vi "daq.vi"(5 "data queue 1":refnum<queue>, 7 "data queue 2":refnum<queue>, 8 "error in":errorcluster, 9 "finished late":bool, 10 "vars runtime":T2[](array[typedef])=[{"t wait"=1000, "t stim"=0, "t square"=0, "t digStimOne"=0, "t digStimTwo"=0, "t rew"=0, "t onset"=10000, "n stim"=0, "n hit"=0, "n miss"=0, "n catch"=0, "n reject"=0, "n false alarm"=0, "stim amp"=0.0, "stim idx"=0, "next temp"=32.0, "catch"=FALSE, "stimulus"=FALSE, "reward given"=FALSE, "penalty given"=FALSE, "lick"=FALSE, "next reward"=FALSE, "penalty"=FALSE, "backlight"=FALSE, "square"=FALSE, "digStimOne"=FALSE, "digStimTwo"=FALSE, "first run?"=TRUE, "timeout"=FALSE, "free reward"=FALSE, "pairing"=FALSE, "d stim"=0, "d square"=0, "n rew"=0, "t penalty"=0}, {"t wait"=1000, "t stim"=0, "t square"=0, "t digStimOne"=0, "t digStimTwo"=0, "t rew"=0, "t onset"=10000, "n stim"=0, "n hit"=0, "n miss"=0, "n catch"=0, "n reject"=0, "n false alarm"=0, "stim amp"=0.0, "stim idx"=0, "next temp"=32.0, "catch"=FALSE, "stimulus"=FALSE, "reward given"=FALSE, "penalty given"=FALSE, "lick"=FALSE, "next reward"=FALSE, "penalty"=FALSE, "backlight"=FALSE, "square"=FALSE, "digStimOne"=FALSE, "digStimTwo"=FALSE, "first run?"=TRUE, "timeout"=FALSE, "free reward"=FALSE, "pairing"=FALSE, "d stim"=0, "d square"=0, "n rew"=0, "t penalty"=0}, {"t wait"=1000, "t stim"=0, "t square"=0, "t digStimOne"=0, "t digStimTwo"=0, "t rew"=0, "t onset"=10000, "n stim"=0, "n hit"=0, "n miss"=0, "n catch"=0, "n reject"=0, "n false alarm"=0, "stim amp"=0.0, "stim idx"=0, "next temp"=32.0, "catch"=FALSE, "stimulus"=FALSE, "reward given"=FALSE, "penalty given"=FALSE, "lick"=FALSE, "next reward"=FALSE, "penalty"=FALSE, "backlight"=FALSE, "square"=FALSE, "digStimOne"=FALSE, "digStimTwo"=FALSE, "first run?"=TRUE, "timeout"=FALSE, "free reward"=FALSE, "pairing"=FALSE, "d stim"=0, "d square"=0, "n rew"=0, "t penalty"=0}, {"t wait"=1000, "t stim"=0, "t square"=0, "t digStimOne"=0, "t digStimTwo"=0, "t rew"=0, "t onset"=10000, "n stim"=0, "n hit"=0, "n miss"=0, "n catch"=0, "n reject"=0, "n false alarm"=0, "stim amp"=0.0, "stim idx"=0, "next temp"=32.0, "catch"=FALSE, "stimulus"=FALSE, "reward given"=FALSE, "penalty given"=FALSE, "lick"=FALSE, "next reward"=FALSE, "penalty"=FALSE, "backlight"=FALSE, "square"=FALSE, "digStimOne"=FALSE, "digStimTwo"=FALSE, "first run?"=TRUE, "timeout"=FALSE, "free reward"=FALSE, "pairing"=FALSE, "d stim"=0, "d square"=0, "n rew"=0, "t penalty"=0}], 11 "task cluster":T1={"AI"="", "AO"="", "DO"="", "DI"="AI"}) -> (0 "error out":errorcluster, 2 "vars runtime":T2[](array[typedef])=[{"t wait"=1000, "t stim"=0, "t square"=0, "t digStimOne"=0, "t digStimTwo"=0, "t rew"=0, "t onset"=10000, "n stim"=0, "n hit"=0, "n miss"=0, "n catch"=0, "n reject"=0, "n false alarm"=0, "stim amp"=0.0, "stim idx"=0, "next temp"=32.0, "catch"=FALSE, "stimulus"=FALSE, "reward given"=FALSE, "penalty given"=FALSE, "lick"=FALSE, "next reward"=FALSE, "penalty"=FALSE, "backlight"=FALSE, "square"=FALSE, "digStimOne"=FALSE, "digStimTwo"=FALSE, "first run?"=FALSE, "timeout"=FALSE, "free reward"=FALSE, "pairing"=FALSE, "d stim"=0, "d square"=0, "n rew"=0, "t penalty"=0}, {"t wait"=1000, "t stim"=0, "t square"=0, "t digStimOne"=0, "t digStimTwo"=0, "t rew"=0, "t onset"=10000, "n stim"=0, "n hit"=0, "n miss"=0, "n catch"=0, "n reject"=0, "n false alarm"=0, "stim amp"=0.0, "stim idx"=0, "next temp"=32.0, "catch"=FALSE, "stimulus"=FALSE, "reward given"=FALSE, "penalty given"=FALSE, "lick"=FALSE, "next reward"=FALSE, "penalty"=FALSE, "backlight"=FALSE, "square"=FALSE, "digStimOne"=FALSE, "digStimTwo"=FALSE, "first run?"=FALSE, "timeout"=FALSE, "free reward"=FALSE, "pairing"=FALSE, "d stim"=0, "d square"=0, "n rew"=0, "t penalty"=0}, {"t wait"=1000, "t stim"=0, "t square"=0, "t digStimOne"=0, "t digStimTwo"=0, "t rew"=0, "t onset"=10000, "n stim"=0, "n hit"=0, "n miss"=0, "n catch"=0, "n reject"=0, "n false alarm"=0, "stim amp"=0.0, "stim idx"=0, "next temp"=32.0, "catch"=FALSE, "stimulus"=FALSE, "reward given"=FALSE, "penalty given"=FALSE, "lick"=FALSE, "next reward"=FALSE, "penalty"=FALSE, "backlight"=FALSE, "square"=FALSE, "digStimOne"=FALSE, "digStimTwo"=FALSE, "first run?"=FALSE, "timeout"=FALSE, "free reward"=FALSE, "pairing"=FALSE, "d stim"=0, "d square"=0, "n rew"=0, "t penalty"=0}, {"t wait"=1000, "t stim"=0, "t square"=0, "t digStimOne"=0, "t digStimTwo"=0, "t rew"=0, "t onset"=10000, "n stim"=0, "n hit"=0, "n miss"=0, "n catch"=0, "n reject"=0, "n false alarm"=0, "stim amp"=0.0, "stim idx"=0, "next temp"=32.0, "catch"=FALSE, "stimulus"=FALSE, "reward given"=FALSE, "penalty given"=FALSE, "lick"=FALSE, "next reward"=FALSE, "penalty"=FALSE, "backlight"=FALSE, "square"=FALSE, "digStimOne"=FALSE, "digStimTwo"=FALSE, "first run?"=FALSE, "timeout"=FALSE, "free reward"=FALSE, "pairing"=FALSE, "d stim"=0, "d square"=0, "n rew"=0, "t penalty"=0}], 3 "task cluster":T1={"AI"="", "AO"="", "DO"="", "DI"="AI"})   [LabVIEW 2016]
uses:
  Type Definitions/data.ctl
  Type Definitions/tasks.ctl
  Type Definitions/vars_runtime.ctl
  <vilib>/DAQmx/read.llb/DAQmx Read (Analog 1D DBL NChan 1Samp).vi
  <vilib>/DAQmx/write.llb/DAQmx Write (Digital 1D Bool NChan 1Samp 1Line).vi
  <vilib>/DAQmx/write.llb/DAQmx Write (Analog 1D DBL NChan 1Samp).vi
  <vilib>/DAQmx/read.llb/DAQmx Read (Digital 1D Bool NChan 1Samp 1Line).vi
  <vilib>/DAQmx/miscellaneous.llb/DAQmx Fill In Error Info.vi
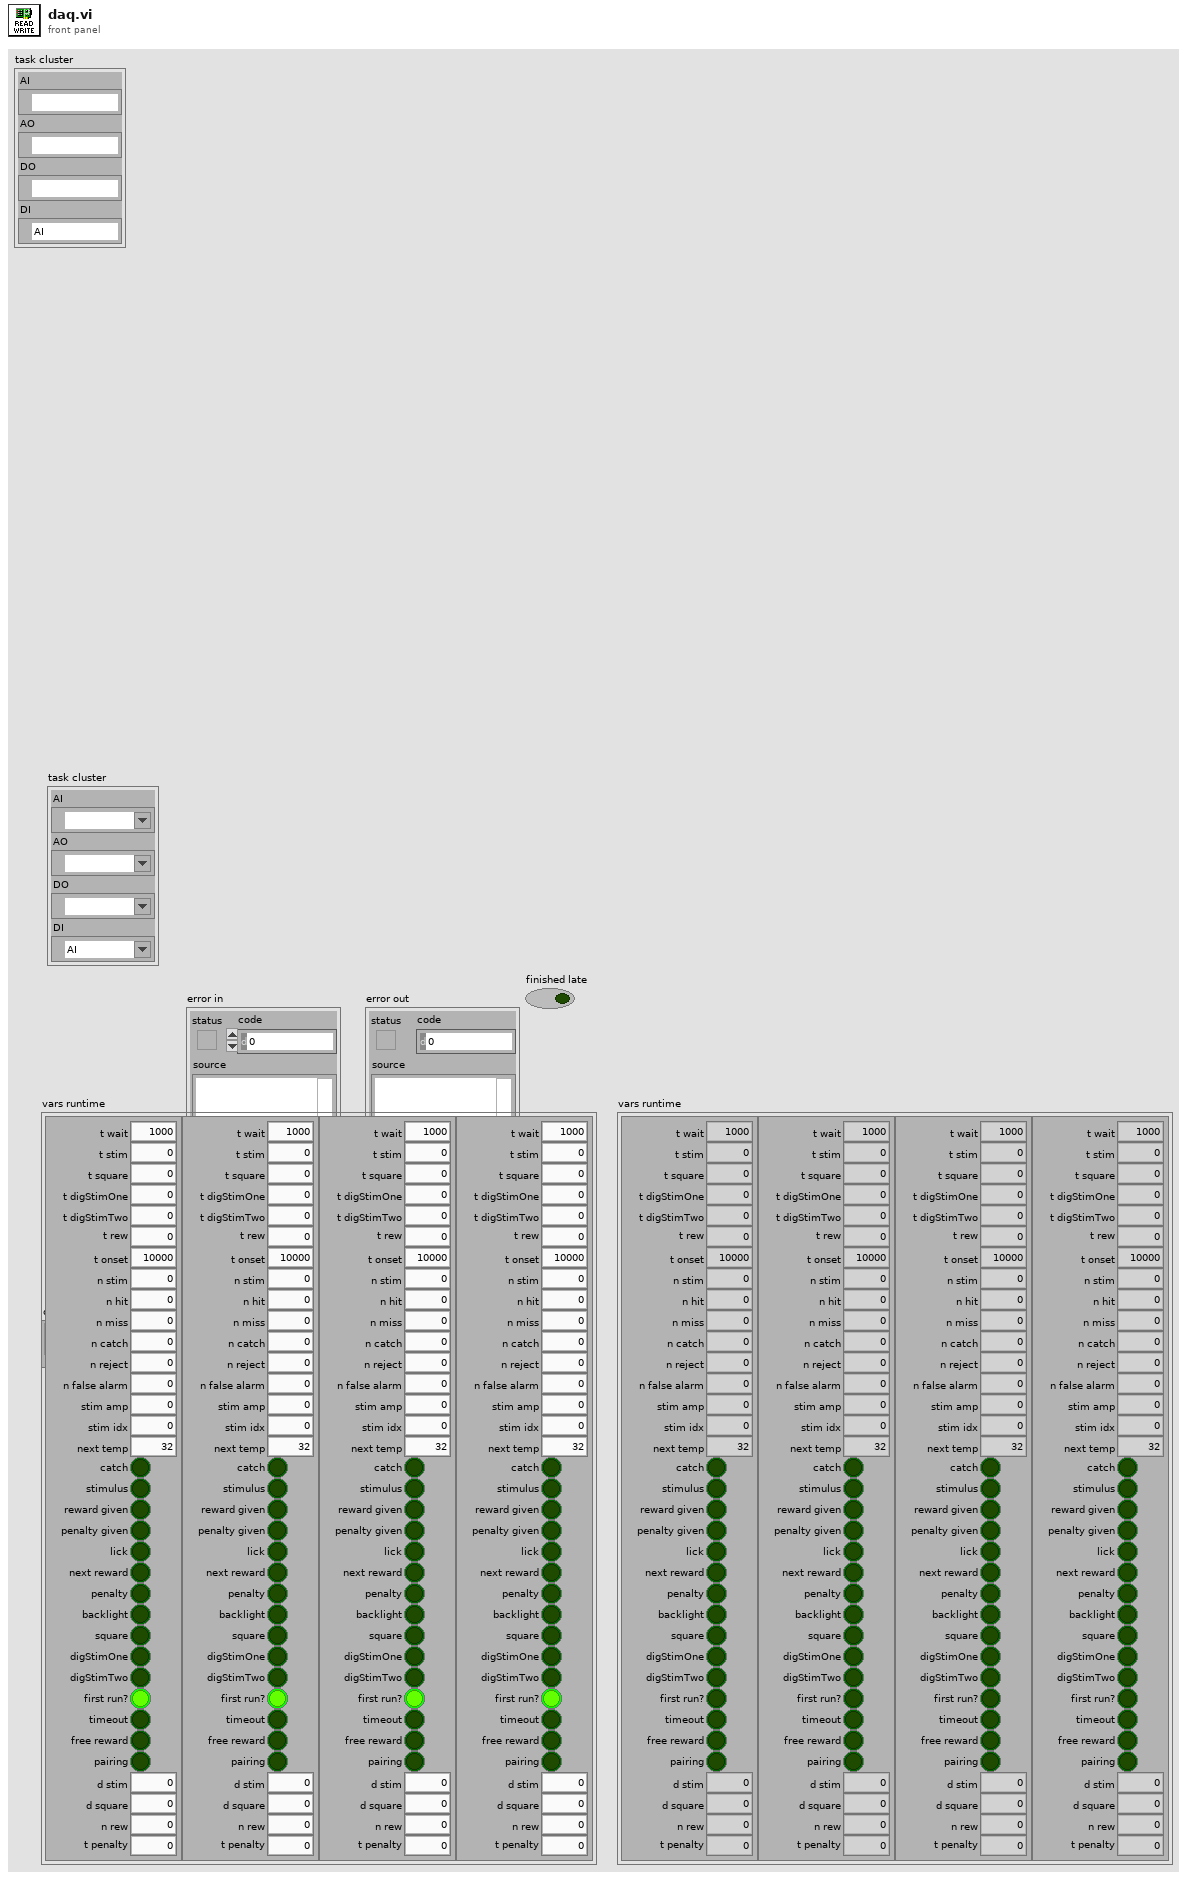
[diagram p1: front panel]
types:
  T1 = typedef "tasks.ctl" = cluster{"AI":refnum<k21>, "AO":refnum<k21>, "DO":refnum<k21>, "DI":refnum<k21>}
  T2 = typedef "vars_runtime.ctl" = cluster{"t wait":u16, "t stim":u16, "t square":u16, "t digStimOne":u16, "t digStimTwo":u16, "t rew":u16, "t onset":u32, "n stim":u16, "n hit":u16, "n miss":u16, "n catch":u16, "n reject":u16, "n false alarm":u16, "stim amp":sgl, "stim idx":i32, "next temp":sgl, "catch":bool, "stimulus":bool, "reward given":bool, "penalty given":bool, "lick":bool, "next reward":bool, "penalty":bool, "backlight":bool, "square":bool, "digStimOne":bool, "digStimTwo":bool, "first run?":bool, "timeout":bool, "free reward":bool, "pairing":bool, "d stim":u16, "d square":u16, "n rew":u16, "t penalty":u16}
  T3 = typedef "data.ctl" = cluster{"time":dbl, "finished late":bool, "temp out":sgl[], "temp in":sgl[], "stim":bool[], "catch":bool[], "lick":bool[], "reward":bool[], "penalty":bool[], "backlight":bool[], "freqstim":bool[], "dStimOne":bool[], "dStimTwo":bool[], "free reward":bool[], "timeout":bool[], "pairing":bool[]}
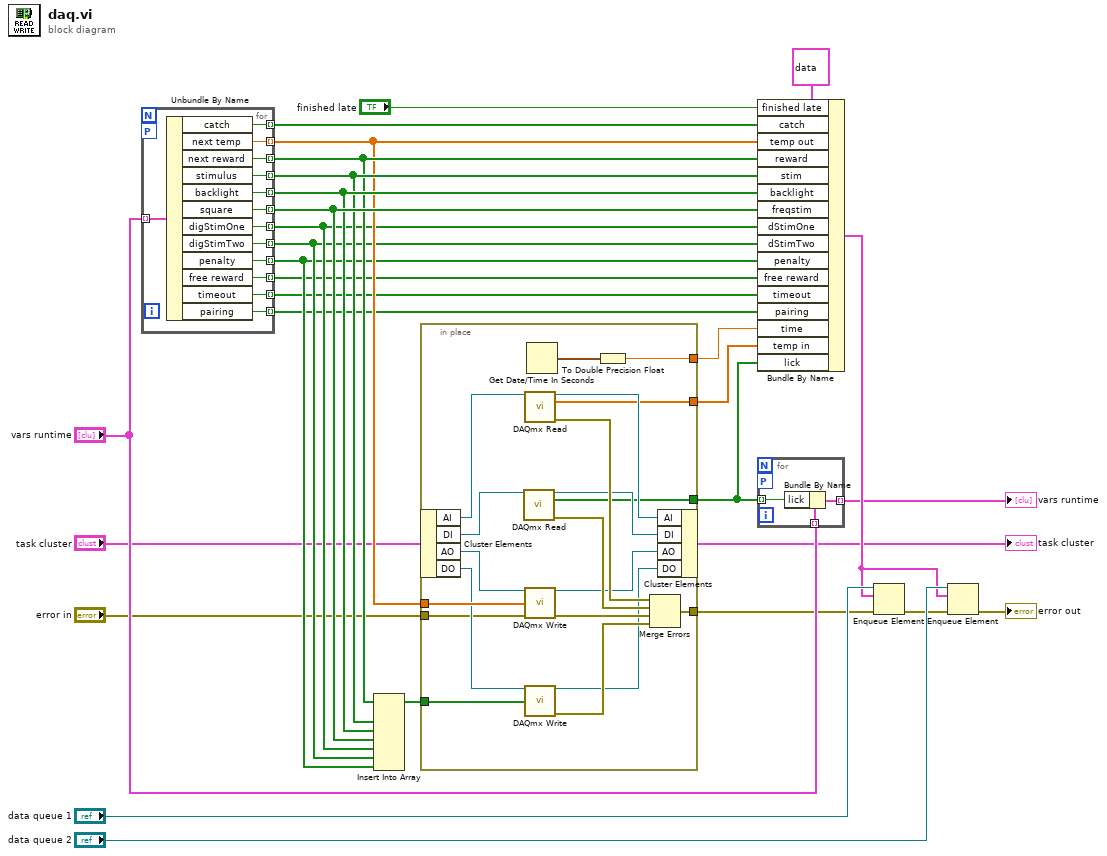
[diagram p0: block diagram]
diagram:
  n1 = for {
    tunnel: "vars runtime" -> [w42] mode=indexing
    tunnel: [w41] -> w26 mode=indexing
    workers-P: _ -> [_]
    tunnel: [w40] -> w27 mode=indexing
    tunnel: [w39] -> w28 mode=indexing
    tunnel: [w38] -> w25 mode=indexing
    tunnel: [w37] -> w10 mode=indexing
    tunnel: [w36] -> w29 mode=indexing
    tunnel: [w35] -> w22 mode=indexing
    tunnel: [w34] -> w6 mode=indexing
    tunnel: [w33] -> w7 mode=indexing
    tunnel: [w32] -> w24 mode=indexing
    tunnel: [w31] -> w23 mode=indexing
    tunnel: [w30] -> w5 mode=indexing
    n2 = Unbundle By Name(w42) -> ("catch"=w37:bool, "next temp"=w38:sgl, "next reward"=w41:bool, "stimulus"=w40:bool, "backlight"=w39:bool, "square"=w36:bool, "digStimOne"=w32:bool, "digStimTwo"=w31:bool, "penalty"=w35:bool, "free reward"=w30:bool, "timeout"=w34:bool, "pairing"=w33:bool)
  }
  n3 = Insert Into Array(array=w26, new element #1=w27, new element #2=w28, new element #3=w29, new element #4=w24, new element #5=w23, new element #6=w22) -> (w12:bool[])  [unwired: 1 in]
  n4 = in-place "Data Acquisition" {
    in-place-border: [w59] -> w14
    in-place-border: w25 -> [w58]
    in-place-border: w12 -> [w57]
    in-place-border: [w49] -> w2
    in-place-border: [w47] -> w19
    in-place-border: "error in" -> [w43]
    in-place-border: [w44] -> w1
    n5 = in-place-cluster #1("task cluster") -> ("AI"=w55:refnum<k21>, "DI"=w46:refnum<k21>, "AO"=w52:refnum<k21>, "DO"=w53:refnum<k21>)
    n6 = call-poly <vilib>:"DAQmx Read.vi"("task/channels in"=w46) -> ("task out"=w45:refnum<k21>, "data"=w44:bool[], "error out"=w60:errorcluster)  [unwired: 12 in]
    n7 = call-poly <vilib>:"DAQmx Read.vi"("task/channels in"=w55) -> ("task out"=w54:refnum<k21>, "data"=w49:dbl[], "error out"=w56:errorcluster)  [unwired: 12 in]
    n8 = call-poly <vilib>:"DAQmx Write.vi"("task/channels in"=w52, "data"=w58, "error in"=w43) -> ("task out"=w50:refnum<k21>, "error out"=w61:errorcluster)  [unwired: 10 in, 1 out]
    n9 = call-poly <vilib>:"DAQmx Write.vi"("task/channels in"=w53, "data"=w57) -> ("task out"=w51:refnum<k21>, "error out"=w62:errorcluster)  [unwired: 11 in, 1 out]
    n10 = Get Date/Time In Seconds() -> (seconds since 1Jan1904=w48:timestamp)
    n11 = To Double Precision Float(number=w48) -> (double precision float=w47:dbl)
    n12 = Merge Errors(w56, w60, w61, w62) -> (w59:errorcluster)
    n13 = in-place-cluster #1("AI"=w54, "DI"=w45, "AO"=w50, "DO"=w51) -> (→"task cluster":T1)
  }
  n14 = Bundle By Name(cluster=T3 {"time"=0.0, "finished late"=FALSE, "temp out"=[], "temp in"=[], "stim"=[FALSE, FALSE, FALSE, FALSE], "catch"=[], "lick"=[FALSE, FALSE, FALSE, FALSE], "reward"=[FALSE, FALSE, FALSE, FALSE], "penalty"=[], "backlight"=[], "freqstim"=[], "dStimOne"=[], "dStimTwo"=[], "free reward"=[], "timeout"=[], "pairing"=[]} ("data cluster"), "finished late"="finished late", "catch"=w10, "temp out"=w25, "reward"=w26, "stim"=w27, "backlight"=w28, "freqstim"=w29, "dStimOne"=w24, "dStimTwo"=w23, "penalty"=w22, "free reward"=w5, "timeout"=w6, "pairing"=w7, "time"=w19, "temp in"=w2, "lick"=w1) -> (w13:T3)
  n15 = for {
    tunnel: [w65] -> w4 mode=indexing
    tunnel: "vars runtime" -> [w64] mode=indexing
    tunnel: w1 -> [w63] mode=indexing
    workers-P: _ -> [_]
    n16 = Bundle By Name(cluster=w64, "lick"=w63) -> (w65:T2)
  }
  "vars runtime" <- w4
  n17 = Enqueue Element(queue="data queue 1", element=w13, error in (no error)=w14) -> (error out=w15:errorcluster)  [unwired: 1 in, 2 out]
  n18 = Enqueue Element(queue="data queue 2", element=w13, error in (no error)=w15) -> (error out=→"error out":errorcluster)  [unwired: 1 in, 2 out]
